vi "원소 큐 2개 데이터 넣기.vi"() -> ()   [LabVIEW 2020]
panel:
  out "원소":dbl[][](array[numeric])
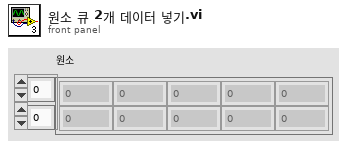
[diagram p1: front panel]
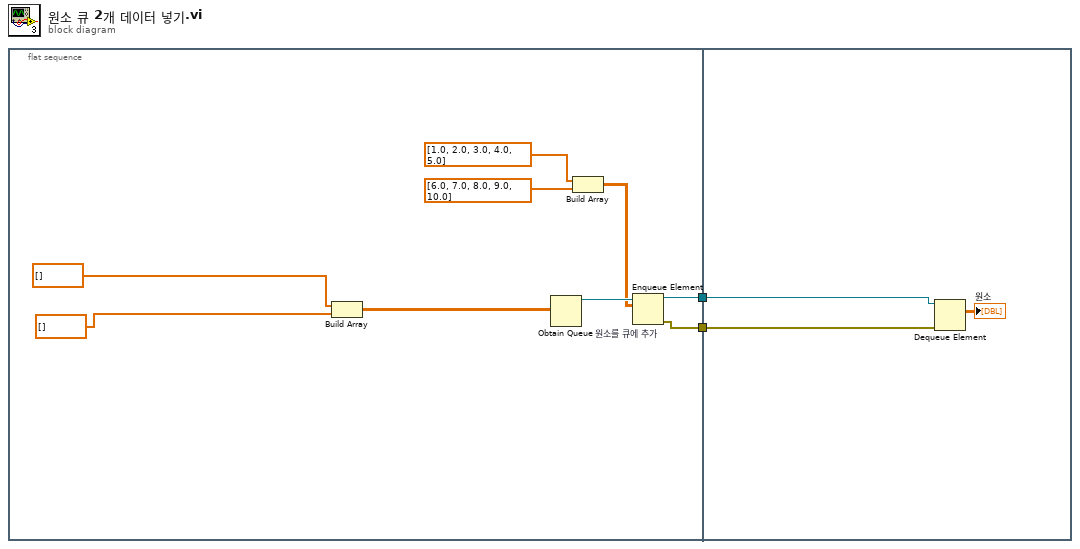
[diagram p0: block diagram]
diagram:
  n1 = flat-sequence {
    tunnel: [w4] -> w2
    tunnel: [w3] -> w1
    tunnel: w2 -> [w14]
    tunnel: w1 -> [w13]
    frame #0 {
      n2 = Build Array(dbl[] [], dbl[] []) -> (w9:dbl[][])
      n3 = Obtain Queue(element data type=w9) -> (queue out=w8:refnum<queue>)  [unwired: 4 in, 2 out]
      n4 = Build Array(dbl[] [1.0, 2.0, 3.0, 4.0, 5.0], dbl[] [6.0, 7.0, 8.0, 9.0, 10.0]) -> (w5:dbl[][])
      n5 = Enqueue Element "원소를 큐에 추가"(queue=w8, element=w5) -> (queue out=w4:refnum<queue>, error out=w3:errorcluster)  [unwired: 2 in, 1 out]
    }
    frame #1 {
      n6 = Dequeue Element(queue=w14, error in (no error)=w13) -> (element=→"원소":dbl[][])  [unwired: 1 in, 3 out]
    }
  }
